vi "RTS Extract Config Data.vi"(8 "Error In":errorcluster, 11 "all rows":string[][](array[string])) -> (0 "Error Out":errorcluster, 3 "Array":string[](array[string]))   [LabVIEW 2016]
uses:
  <vilib>/Utility/error.llb/whitespace.ctl
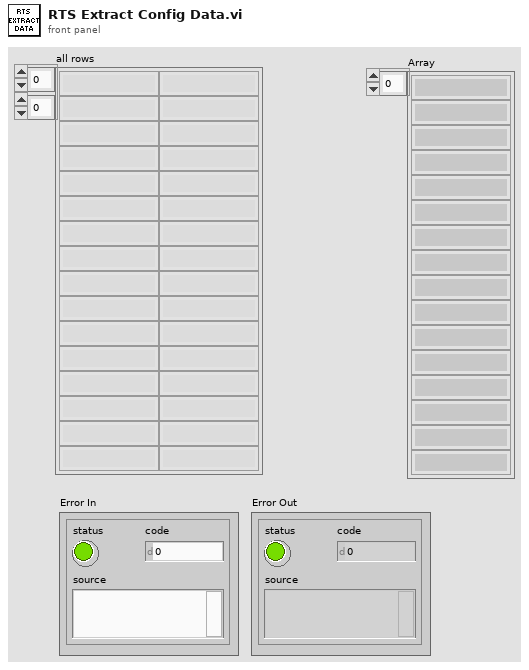
[diagram p1: front panel]
types:
  T1 = typedef "whitespace.ctl" = u16
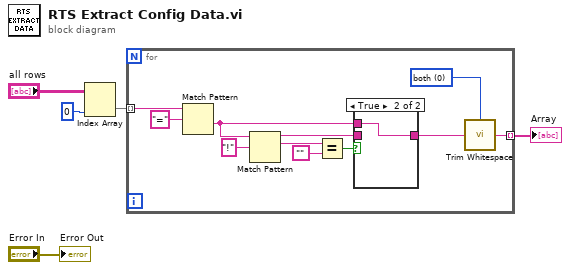
[diagram p0: block diagram]
diagram:
  n1 = Index Array(array="all rows", index (col)=0 ("disabled index (col)")) -> (element=w4:string[])  [unwired: 1 in]
  n2 = for {
    tunnel: w4 -> [w15] mode=indexing
    tunnel: [w7] -> w5 mode=indexing
    w6 = T1 0 items=["both", "start of string", "end of string"] ("location (both)")
    n3 = Match Pattern(string=w15, regular expression="=") -> (after substring=w11:string)  [unwired: 1 in, 3 out]
    n4 = Match Pattern(string=w11, regular expression="!") -> (before substring=w9:string, match substring=w13:string)  [unwired: 1 in, 2 out]
    n5 = Equal?(x=w13, y="") -> (x = y?=w10:bool)
    n6 = case shown="True" w10 {
      tunnel: w11 -> [_ w18]
      tunnel: [w17 w18] -> w8
      tunnel: w9 -> [w17 _]
      frame False {
      }
      frame True {
      }
    }
    n7 = call <vilib>:"Trim Whitespace.vi"("string"=w8, "location (both)"=w6) -> ("trimmed string"=w7:string)
  }
  "Array" <- w5
  "Error Out" <- "Error In"
